vi "NumEntry.vi"() -> (2 "Current Value":dbl format="%#.0f")   [LabVIEW 2018]
doc: "This VI takes the control reference for a digital numeric indicator and provides a calculator style keypad for number entry. The reference is double, but it only works for positive, integer values"
panel:
  in  "Value":dbl
  in  "Enter":bool
  in  "Button 0":bool
  in  "Button 9":bool
  in  "Button 8":bool
  in  "Button 7":bool
  in  "Button 6":bool
  in  "Button 5":bool
  in  "Button 4":bool
  in  "Button 3":bool
  in  "CLR":bool
  in  "BS":bool
  in  "Cancel":bool
  in  "Button 2":bool
  in  "Button 1":bool
  in  "New Value":dbl format="%#.0f"
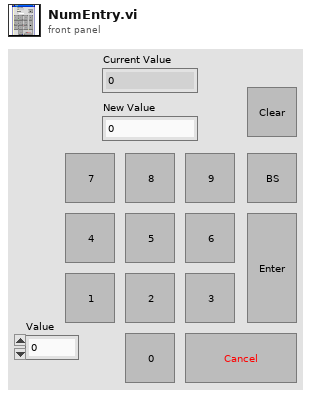
[diagram p1: front panel]
types:
  T1 = typedef "LVMinMaxIncTypeDef.ctl" = cluster{"Minimum":dbl, "Maximum":dbl, "Increment":dbl}
  T2 = typedef "LVOutOfRangeActionTypeDef.ctl" = cluster{"OutOfRngActMin":u8, "OutOfRngActMax":u8, "OutOfRngActInc":u8}
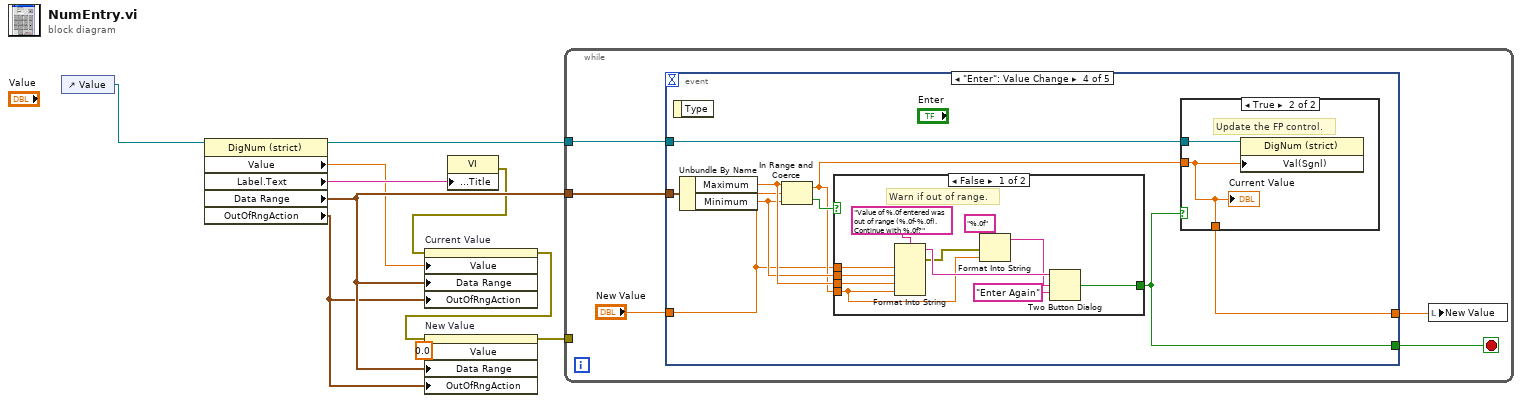
[diagram p0: block diagram]
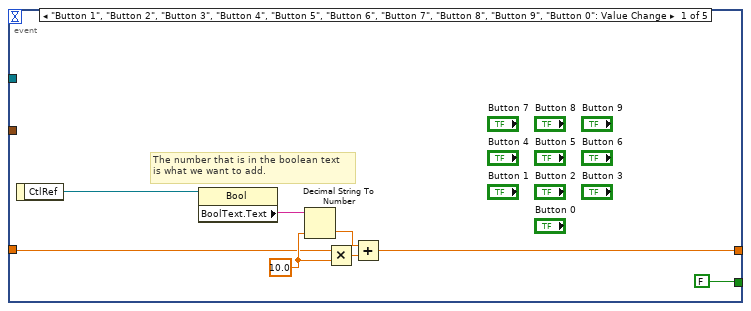
[diagram p2: hidden frame]
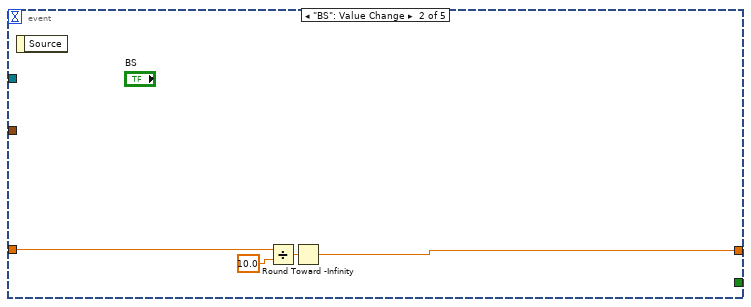
[diagram p3: hidden frame]
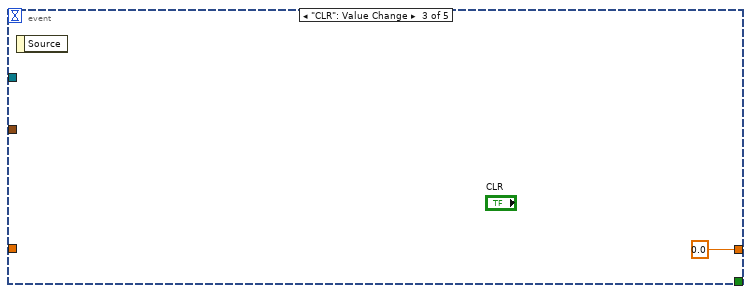
[diagram p4: hidden frame]
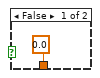
[diagram p5: hidden frame]
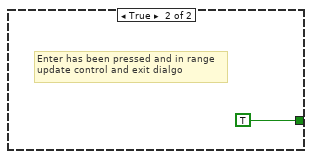
[diagram p6: hidden frame]
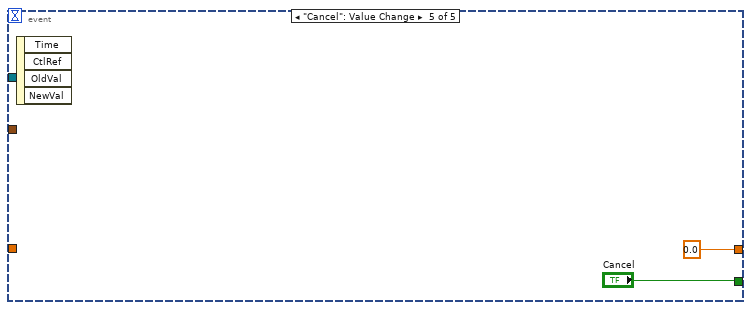
[diagram p7: hidden frame]
diagram:
  n1 = control-ref of="Value"() -> (w1:refnum<vi>)
  n2 = property class="DigNum (strict)"(reference=w1) -> (reference out=w9:refnum<vi>, "Value"=w7:dbl, "Label.Text"=w8:string, "Data Range"=w10:T1, "OutOfRngAction"=w5:T2)  [unwired: 1 in, 1 out]
  n3 = property class="VI"("Front Panel.Title"=w8) -> (error out=w3:errorcluster)  [unwired: 2 in, 1 out]
  n4 = property on="Current Value" class="DigNum (strict)"(error in=w3, "Value"=w7, "Data Range"=w10, "OutOfRngAction"=w5) -> (error out=w4:errorcluster)  [unwired: 1 in, 1 out]
  n5 = property on="New Value" class="DigNum (strict)"(error in=w4, "Value"=0.0 ("New Value"), "Data Range"=w10, "OutOfRngAction"=w5) -> (error out=w2:errorcluster)  [unwired: 1 in, 1 out]
  n6 = while {
    tunnel: w10 -> [w12]
    tunnel: w9 -> [w11]
    tunnel: w2 -> [_]
    stop <- w13 stop-if-true
    n7 = event shown="[3] \"Enter\": Value Change" {
      selector: _ -> [_ _ _ _ _]
      dyn-events: _ -> [_ _ _ _ _]
      timeout: _ -> [_ _ _ _ _]
      tunnel: "New Value" -> [w16 w24 _ w30 _]
      tunnel: [w18 w25 0.0 w29 0.0] -> w14
      tunnel: [FALSE _ _ w31 "Cancel"] -> w13
      tunnel: w12 -> [_ _ _ w34 _]
      tunnel: w11 -> [_ _ _ w32 _]
      event "Button 1", "Button 2", "Button 3", "Button 4", "Button 5", "Button 6", "Button 7", "Button 8", "Button 9", "Button 0": Value Change {
        w23 = 10.0 ("y")
        # "The number that is in the boolean text\nis what we want to add."
        n8 = event-data() -> ("CtlRef"=w19:refnum<vi>)  [unwired: 1 out]
        n9 = property class="Bool"(reference=w19) -> ("BoolText.Text"=w21:string)  [unwired: 1 in, 2 out]
        n10 = Decimal String To Number(string=w21, default (0L)=w23) -> (number=w22:dbl)  [unwired: 2 out]
        n11 = Multiply(x=w16, y=w23) -> (x*y=w20:dbl)
        n12 = Add(x=w22, y=w20) -> (x+y=w18:dbl)
      }
      event "BS": Value Change {
        n13 = event-data() -> ()  [unwired: 2 out]
        n14 = Divide(x=w24, y=10.0) -> (x/y=w27:dbl)
        n15 = Round Toward -Infinity(1:w27) -> (0:w25:dbl)
      }
      event "CLR": Value Change {
        n16 = event-data() -> ()  [unwired: 2 out]
      }
      event "Enter": Value Change {
        n17 = event-data() -> ()  [unwired: 2 out]
        n18 = Unbundle By Name(w34) -> ("Maximum"=w36:dbl, "Minimum"=w35:dbl)
        n19 = In Range and Coerce(upper limit=w36, x=w30, lower limit=w35) -> (coerced(x)=w33:dbl, In Range?=w37:bool)
        n20 = case shown="False" w37 {
          tunnel: [w51 TRUE] -> w31
          tunnel: w36 -> [w49 _]
          tunnel: w35 -> [w47 _]
          tunnel: w33 -> [w45 _]
          tunnel: w30 -> [w41 _]
          frame False {
            # "Warn if out of range."
            n21 = Format Into String(format string="Value of %.0f entered was out of range (%.0f-%.0f).  Continue with %.0f?", w41, w47, w49, w45) -> (resulting string=w50:string, error out=w43:errorcluster)  [unwired: 2 in]
            n22 = Format Into String(format string="%.0f", error in=w43, w45) -> (resulting string=w44:string)  [unwired: 1 in, 1 out]
            n23 = Two Button Dialog(message=w50, 1:"Enter Again" ("F button name (\"Cancel\")"), 2:w44) -> (T button?=w51:bool)
          }
          frame True {
            # "Enter has been pressed and in range\nupdate control and exit dialgo"
          }
        }
        n24 = case shown="True" w31 {
          tunnel: w32 -> [_ w40]
          tunnel: w33 -> [_ w39]
          tunnel: [0.0 ("Maximum") w39] -> w29
          frame False {
          }
          frame True {
            # "Update the FP control."
            n25 = property class="DigNum (strict)"(reference=w40, "Val(Sgnl)"=w39) -> ()  [unwired: 1 in, 2 out]
            "Current Value" <- w39
          }
        }
      }
      event "Cancel": Value Change {
        n26 = event-data() -> ()  [unwired: 5 out]
      }
    }
    n27 = local write "New Value"(w14) -> ()
  }
